vi "Get Non-Qualified Name.vi"(10 "VI Name":string) -> (2 "Non-Qualified VI Name":string)   [LabVIEW 2020]
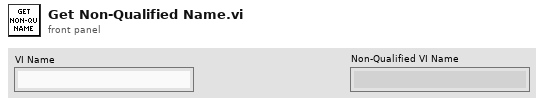
[diagram p1: front panel]
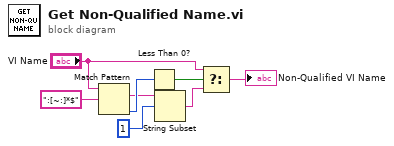
[diagram p0: block diagram]
diagram:
  n1 = Match Pattern(string="VI Name", regular expression=":[~:]*$") -> (match substring=w5:string, offset past match=w8:i32)  [unwired: 3 out]
  n2 = Less Than 0?(x=w8) -> (x < 0?=w4:bool)
  n3 = String Subset(string=w5, offset (0)=1) -> (substring=w2:string)  [unwired: 1 out]
  n4 = Select(t="VI Name", s=w4, f=w2) -> (s? t:f=→"Non-Qualified VI Name":string)
